vi "PinholesSingle.vi"(4 "Current Threshold [nA]":dbl, 6 "Channel":i32) -> (0 "Compliance?":bool, 1 "channel excluded":bool, 2 "Current [nA]":dbl, 3 "Flag":i32)   [LabVIEW 2019]
uses:
  general_VIs/globals/QC_MeasurementSetup.vi
  InstrControl/Switching/Switching.lvclass
  InstrControl/SupplyControl/SupplyControl.lvclass
panel:
  in  "settling\ndelay":i32
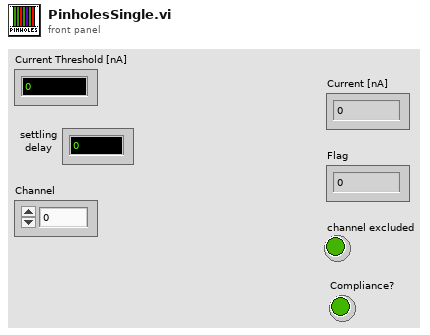
[diagram p1: front panel]
types:
  T1 = cluster{"Bias Supply":refnum<class "SupplyControl.lvclass">, "SMU":refnum<class "SupplyControl.lvclass">, "LCR":refnum<class "LCRControl.lvclass">, "Probe Card Channels":i32, "Bias Voltage [V]":dbl, "First strip":i32, "Last strip":i32, "Base Voltage [V]":dbl, "Base Ramp Step [V]":dbl, "Base Ramp Interval [ms]":u32, "High Voltage [V]":dbl, "High Ramp Step [V]":dbl, "High Ramp Interval [ms]":u32, "AC frequency [Hz]":i32, "AC amplitude [V]":dbl, "RC Configuration":u16, "Single Needle":bool, "Temperature Readout":enum16{"Read Arduino", "Enter manually"}, "Arduino":refnum<class "ArduinoControl.lvclass">, "Fraction of good strips [%]":dbl, "ProbeStation":refnum<class "ProbeStationControl.lvclass">, "Switching":refnum<class "Switching.lvclass">, "Matrix used?":bool, "Matrix X Channels":cluster{"Bias Supply / SMU LO":i32, "Bias Supply / SMU HI":i32, "CV Box LO":i32, "CV Box HI":i32, "CV Box LO IN":i32, "CV Box HI IN":i32, "Volt meter LO":i32, "Volt meter HI":i32, "Mux1 C1":i32, "Mux1 C2":i32, "Mux2 C1":i32, "Mux2 C2":i32}, "Pinholes Y/N":bool, "Capacitance Y/N":bool, "Resistance Y/N":bool, "Bias Supply Name":string, "SMU Name":string, "LCR Name":string}
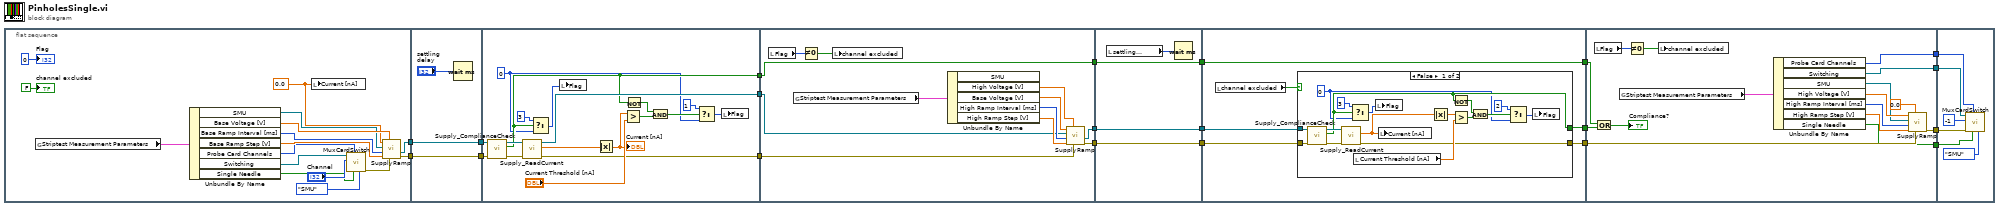
[diagram p0: block diagram]
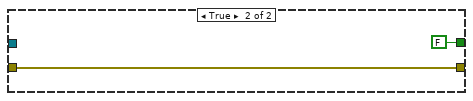
[diagram p2: hidden frame]
diagram:
  n1 = flat-sequence {
    tunnel: [w28] -> w14
    tunnel: [w27] -> w12
    tunnel: [w38] -> w15
    tunnel: w14 -> [w38]
    tunnel: [w37] -> w13
    tunnel: w12 -> [w37]
    tunnel: [w46] -> w20
    tunnel: w15 -> [w50]
    tunnel: w13 -> [w49]
    tunnel: [w48] -> w11
    tunnel: [w47] -> w10
    tunnel: w20 -> [w69]
    tunnel: [w69] -> w17
    tunnel: w11 -> [w63]
    tunnel: w10 -> [w62]
    tunnel: [w61] -> w8
    tunnel: [w60] -> w4
    tunnel: w17 -> [w73]
    tunnel: [w73] -> w16
    tunnel: [w71] -> w9
    tunnel: w8 -> [w71]
    tunnel: [w70] -> w5
    tunnel: w4 -> [w70]
    tunnel: w16 -> [w79]
    tunnel: [w79] -> w19
    tunnel: [w78] -> w18
    tunnel: w9 -> [w76]
    tunnel: [w75] -> w7
    tunnel: w5 -> [w74]
    tunnel: w19 -> [w103]
    tunnel: w18 -> [w102]
    tunnel: w7 -> [w108]
    tunnel: [w107] -> w6
    tunnel: [w101] -> w3
    tunnel: [w100] -> w2
    tunnel: [w99] -> w1
    tunnel: w6 -> [w119]
    tunnel: w3 -> [w118]
    tunnel: w2 -> [w117]
    tunnel: w1 -> [w116]
    frame #0 {
      w30 = 0.0 ("Starting Voltage")
      n2 = global read "QC_MeasurementSetup.vi" "Striptest Measurement Parameters"() -> (w31:T1)
      n3 = Unbundle By Name(w31) -> ("SMU"=w26:refnum<class "SupplyControl.lvclass">, "Base Voltage [V]"=w32:dbl, "Base Ramp Interval [ms]"=w33:u32, "Base Ramp Step [V]"=w34:dbl, "Probe Card Channels"=w22:i32, "Switching"=w23:refnum<class "Switching.lvclass">, "Single Needle"=w24:bool)
      n4 = local write "Current [nA]"(w30) -> ()
      n5 = call-dynamic "MuxCardSwitch.vi"("Instrument"=enum16{"SMU", "LCR"}."SMU", "Single Needle"=w24, "Probe Card Channels"=w22, "Switch to channel"="Channel", "Switching in"=w23) -> ("error out"=w29:errorcluster)  [unwired: 4 in, 2 out]
      n6 = call "SupplyRamp.vi"("error in"=w29, "Requested Voltage"=w32, "Step Size"=w34, "Step Delay"=w33, "Supply IN"=w26, "Starting Voltage"=w30) -> ("error out"=w28:errorcluster, "Supply OUT"=w27:refnum<class "SupplyControl.lvclass">)  [unwired: 2 in, 2 out]
      "Flag" <- 0
      "channel excluded" <- FALSE
    }
    frame #1 {
      n7 = Wait (ms)(milliseconds to wait="settling\ndelay") -> ()  [unwired: 1 out]
    }
    frame #2 {
      w40 = 0
      n8 = call-dynamic "Supply_ComplianceCheck.vi"("error in (no error)"=w50, "SupplyControl in"=w49) -> ("error out"=w52:errorcluster, "Compliance exceeded?"=w46:bool, "SupplyControl out"=w53:refnum<class "SupplyControl.lvclass">)  [unwired: 6 in, 1 out]
      n9 = call-dynamic "Supply_ReadCurrent.vi"("error in (no error)"=w52, "SupplyControl in"=w53) -> ("error out"=w47:errorcluster, "Current in nA"=w57:dbl, "SupplyControl out"=w48:refnum<class "SupplyControl.lvclass">)  [unwired: 7 in]
      n10 = Select(t=3, s=w46, f=w40) -> (s? t:f=w45:i32)
      n11 = local write "Flag"(w45) -> ()
      n12 = Absolute Value(x=w57) -> (abs(x)=w51:dbl)
      "Current [nA]" <- w51
      n13 = Greater?(x=w51, y="Current Threshold [nA]") -> (0:w54:bool)
      n14 = Not(x=w46) -> (.not. x?=w55:bool)
      n15 = And(x=w55, y=w54) -> (x .and. y?=w43:bool)
      n16 = Select(t=1, s=w43, f=w40) -> (s? t:f=w42:i32)
      n17 = local write "Flag"(w42) -> ()
    }
    frame #3 {
      n18 = local read "Flag"() -> (w58:i32)
      n19 = global read "QC_MeasurementSetup.vi" "Striptest Measurement Parameters"() -> (w65:T1)
      n20 = Not Equal To 0?(x=w58) -> (x != 0?=w59:bool)
      n21 = local write "channel excluded"(w59) -> ()
      n22 = Unbundle By Name(w65) -> ("High Voltage [V]"=w64:dbl, "Base Voltage [V]"=w68:dbl, "High Ramp Interval [ms]"=w67:u32, "High Ramp Step [V]"=w66:dbl)  [unwired: 1 out]
      n23 = call "SupplyRamp.vi"("error in"=w62, "Requested Voltage"=w64, "Step Size"=w66, "Step Delay"=w67, "Supply IN"=w63, "Starting Voltage"=w68) -> ("error out"=w61:errorcluster, "Supply OUT"=w60:refnum<class "SupplyControl.lvclass">)  [unwired: 2 in, 2 out]
    }
    frame #4 {
      n24 = local read "settling\ndelay"() -> (w72:i32)
      n25 = Wait (ms)(milliseconds to wait=w72) -> ()  [unwired: 1 out]
    }
    frame #5 {
      n26 = local read "channel excluded"() -> (w77:bool)
      n27 = case shown="False" w77 {
        tunnel: [w81 FALSE] -> w78
        tunnel: w76 -> [w89 w97]
        tunnel: [w88 w97] -> w75
        tunnel: w74 -> [w87 _]
        frame False {
          w80 = 0
          n28 = call-dynamic "Supply_ComplianceCheck.vi"("error in (no error)"=w89, "SupplyControl in"=w87) -> ("error out"=w90:errorcluster, "Compliance exceeded?"=w81:bool, "SupplyControl out"=w91:refnum<class "SupplyControl.lvclass">)  [unwired: 6 in, 1 out]
          n29 = call-dynamic "Supply_ReadCurrent.vi"("error in (no error)"=w90, "SupplyControl in"=w91) -> ("error out"=w88:errorcluster, "Current in nA"=w96:dbl)  [unwired: 7 in, 1 out]
          n30 = Select(t=3, s=w81, f=w80) -> (s? t:f=w84:i32)
          n31 = local read "Current Threshold [nA]"() -> (w93:dbl)
          n32 = local write "Flag"(w84) -> ()
          n33 = local write "Current [nA]"(w96) -> ()
          n34 = Absolute Value(x=w96) -> (abs(x)=w92:dbl)
          n35 = Not(x=w81) -> (.not. x?=w95:bool)
          n36 = Greater?(x=w92, y=w93) -> (0:w94:bool)
          n37 = And(x=w95, y=w94) -> (x .and. y?=w82:bool)
          n38 = Select(t=2, s=w82, f=w80) -> (s? t:f=w83:i32)
          n39 = local write "Flag"(w83) -> ()
        }
        frame True {
        }
      }
    }
    frame #6 {
      n40 = local read "Flag"() -> (w105:i32)
      n41 = Or(x=w103, y=w102) -> (x .or. y?=→"Compliance?":bool)
      n42 = global read "QC_MeasurementSetup.vi" "Striptest Measurement Parameters"() -> (w110:T1)
      n43 = Not Equal To 0?(x=w105) -> (x != 0?=w106:bool)
      n44 = local write "channel excluded"(w106) -> ()
      n45 = Unbundle By Name(w110) -> ("Probe Card Channels"=w100:i32, "Switching"=w101:refnum<class "Switching.lvclass">, "SMU"=w111:refnum<class "SupplyControl.lvclass">, "High Voltage [V]"=w114:dbl, "High Ramp Interval [ms]"=w113:u32, "High Ramp Step [V]"=w112:dbl, "Single Needle"=w99:bool)
      n46 = call "SupplyRamp.vi"("error in"=w108, "Requested Voltage"=0.0, "Step Size"=w112, "Step Delay"=w113, "Supply IN"=w111, "Starting Voltage"=w114) -> ("error out"=w107:errorcluster)  [unwired: 2 in, 3 out]
    }
    frame #7 {
      n47 = call-dynamic "MuxCardSwitch.vi"("Instrument"=enum16{"SMU", "LCR"}."SMU", "Single Needle"=w116, "Probe Card Channels"=w117, "error in (no error)"=w119, "Switch to channel"=-1, "Switching in"=w118) -> ()  [unwired: 3 in, 3 out]
    }
  }
